vi "RT.vi"() -> ()   [LabVIEW 2017]
uses:
  <vilib>/Instr/_visa.llb/VISA Configure Serial Port (Instr).vi
panel:
  out "error out":errorcluster
  out "1":u32
  out "0":u32
  out "unsigned byte array":u8[](array[numeric])
  out "read buffer":string
  in  "stop":bool
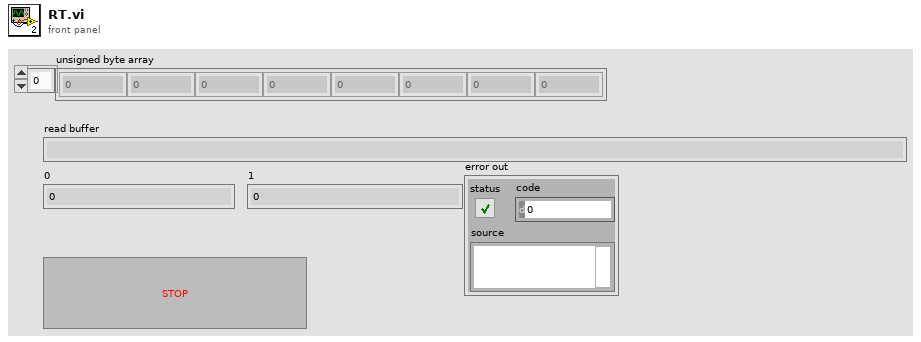
[diagram p1: front panel]
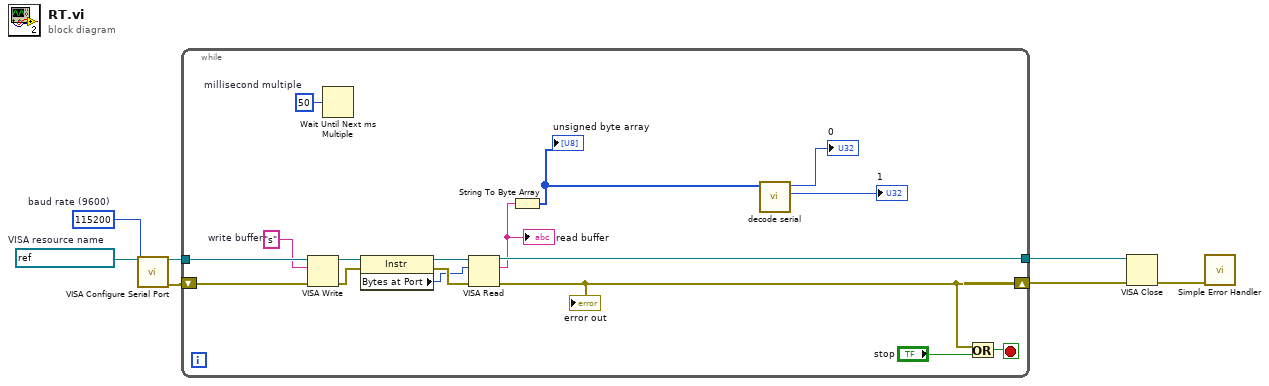
[diagram p0: block diagram]
diagram:
  w1 = u32 115200  # baud rate (9600)
  w5 = refnum<visa-resource-name> "ASRL2::INSTR"  # VISA resource name
  n1 = call-poly "VISA Configure Serial Port"("VISA resource name"=w5, "baud rate (9600)"=w1) -> ("VISA resource name out"=w7:refnum<visa-resource-name>, "error out"=w6:errorcluster)  [unwired: 12 in]
  n2 = while {
    shift-right: [w19] -> w4
    shift-left: w6 -> [w23]
    tunnel: w7 -> [w24]
    tunnel: [w18] -> w3
    stop <- w20 stop-if-true
    w17 = u32 50  # millisecond multiple
    w22 = "s"  # write buffer
    n3 = VISA Write(VISA resource name=w24, write buffer=w22, error in (no error)=w23) -> (VISA resource name out=w15:refnum<visa-resource-name>, error out=w14:errorcluster)  [unwired: 1 out]
    n4 = Wait Until Next ms Multiple(millisecond multiple=w17) -> ()  [unwired: 1 out]
    n5 = property class="Instr"(reference=w15, error in=w14) -> (reference out=w13:refnum<visa-resource-name>, error out=w12:errorcluster, "Bytes at Port"=w8:u32)
    n6 = VISA Read(VISA resource name=w13, byte count=w8, error in (no error)=w12) -> (VISA resource name out=w18:refnum<visa-resource-name>, read buffer=w16:string, error out=w19:errorcluster)  [unwired: 1 out]
    "read buffer" <- w16
    "error out" <- w19
    n7 = String To Byte Array(string=w16) -> (unsigned byte array=w11:u8[])
    "unsigned byte array" <- w11
    n8 = call "decode serial.vi"("unsigned byte array"=w11) -> ("1"=→"1":u32, "0"=→"0":u32)  [unwired: 9 in]
    n9 = Or(x=w19, y="stop") -> (x .or. y?=w20:bool)
  }
  n10 = VISA Close(VISA resource name=w3, error in (no error)=w4) -> (error out=w2:errorcluster)
  n11 = call <vilib>:"Simple Error Handler.vi"("error in (no error)"=w2) -> ()  [unwired: 4 in, 5 out]
